vi "单路通断器（I32).vi"(1 "默认值":i32=-1 format="%.0x", 2 "直通？":bool=TRUE, 3 "X_In":i32) -> (0 "X_Out":i32)   [LabVIEW 2012]
doc: "功能：\n\n返回一个枚举，表明输入数的范围，用于三段比较。\n\n\nCSXCS_366创建。"
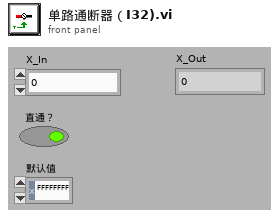
[diagram p1: front panel]
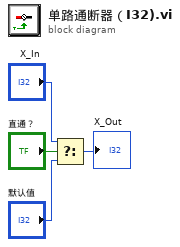
[diagram p0: block diagram]
diagram:
  n1 = Select(t="X_In", s="直通？", f="默认值") -> (s? t:f=→"X_Out":i32)
